vi "430_TCP_Command.vi"(3 "error in (no error)":errorcluster, 4 "Timeout":i32=1000, 5 "Command":string, 6 "connection ID":refnum<k5>) -> (0 "error out":errorcluster, 1 "bytes written":i32, 2 "connection ID out":refnum<k5>)   [LabVIEW 2017]
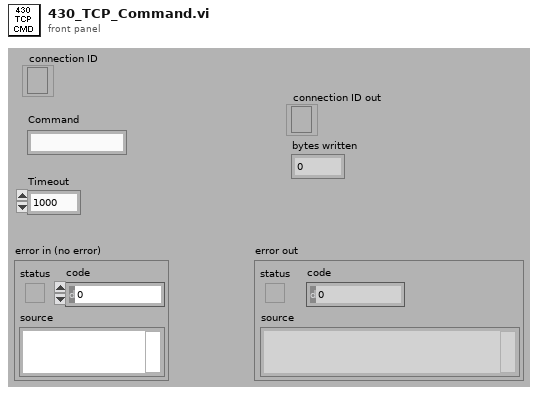
[diagram p1: front panel]
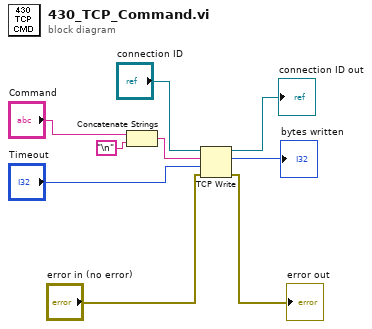
[diagram p0: block diagram]
diagram:
  n1 = Concatenate Strings("Command", "\n") -> (w3:string)
  n2 = TCP Write(connection ID="connection ID", data in=w3, error in (no error)="error in (no error)", 9:"Timeout") -> (connection ID out=→"connection ID out":refnum<k5>, bytes written=→"bytes written":i32, error out=→"error out":errorcluster)
